vi "create_control.vi"(6 "wait for reply (T)":bool=TRUE, 7 "constant":bool, 8 "error in":errorcluster, 9 "terminal_index":i32, 10 "object_id":i32) -> (0 "error out":errorcluster, 1 "timed out?":bool, 3 "created_object_id":i32)   [LabVIEW 2025, in "Scripting Server.lvlib"]
doc: "Creates a control or indicator on the terminal specified by Object ID and Terminal Index, depending on if it's a in- or output of the node. If Constant is set to True, it can only be used on node inputs and will create a constant.\nIt will return the reference to the created control or indicator, that is a reference to the frontpanel element. If constant is True it returns a reference to the block diagram object (constant).\nWhen creating a control or constant you can pass a value to be written to that element."
uses:
  Scripting Server.lvlib
  create_control Argument--cluster.ctl
  create_control (Reply Payload)--cluster.ctl
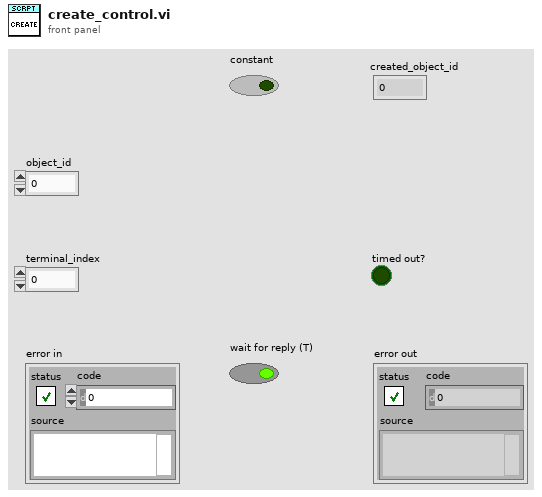
[diagram p1: front panel]
types:
  T1 = typedef "Scripting Server.lvlib/create_control Argument--cluster.ctl" = cluster{"Object ID":i32, "Terminal Index":i32, "Constant":bool, "Wait Notifier":refnum<notifier>, "wait for reply":bool, "Value":string}
  T2 = typedef "Scripting Server.lvlib/Request Events--cluster.ctl" = cluster{"Stop Module":refnum<user-event>, "Show Panel":refnum<user-event>, "Hide Panel":refnum<user-event>, "Get Module Execution Status":refnum<user-event>, "Show Diagram":refnum<user-event>, "New VI":refnum<user-event>, "Add Object":refnum<user-event>, "Connect Objects":refnum<user-event>, "Get Object Terminals":refnum<user-event>, "get vi error list":refnum<user-event>, "Cleanup VI":refnum<user-event>, "create_control":refnum<user-event>, "Run VI":refnum<user-event>, "add_to_selection":refnum<user-event>, "clear_selection_list":refnum<user-event>, "remove_from_selection":refnum<user-event>, "enclose_selection":refnum<user-event>}
  T3 = typedef "Scripting Server.lvlib/create_control (Reply Payload)--cluster.ctl" = cluster{"Object ID":i32, "error":errorcluster}
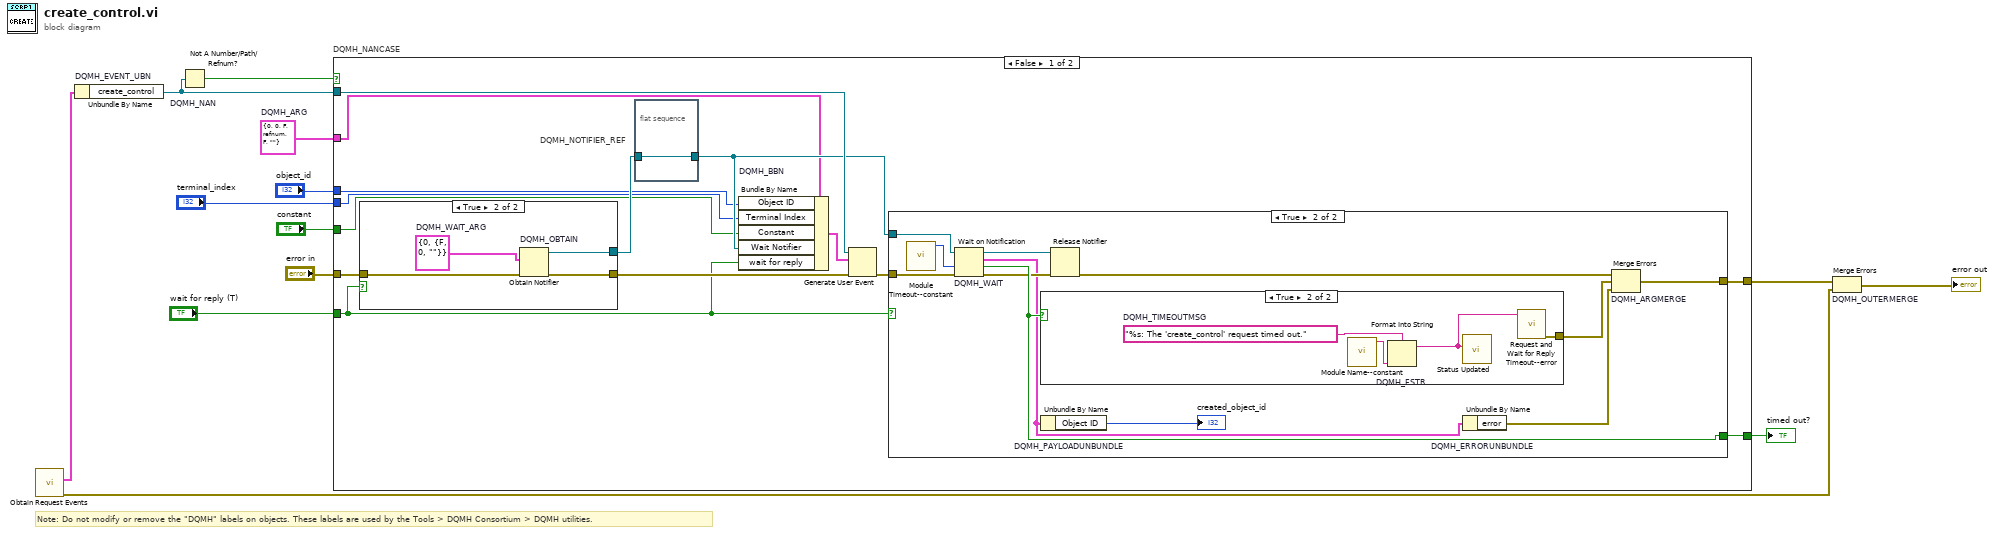
[diagram p0: block diagram]
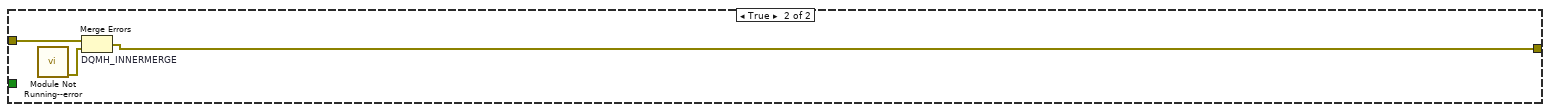
[diagram p5: hidden frame]
diagram:
  w7 = T1 {"Object ID"=0, "Terminal Index"=0, "Constant"=FALSE, "Wait Notifier"=refnum, "wait for reply"=FALSE, "Value"=""}  # DQMH_ARG
  # "Note: Do not modify or remove the \"DQMH\" labels on objects. These labels are used by the Tools > DQMH Consortium > DQMH utilities."
  n1 = call "Obtain Request Events.vi"() -> ("error out"=w2:errorcluster, "Scripting Server Request Events"=w1:T2)  [unwired: 10 in]
  n2 = Unbundle By Name "DQMH_EVENT_UBN"(w1) -> ("create_control"=w11:refnum<user-event>)
  n3 = Not A Number/Path/Refnum? "DQMH_NAN"(number/path/refnum=w11) -> (NaN/Path/Refnum?=w10:bool)
  n4 = case "DQMH_NANCASE" shown="False" w10 {
    tunnel: "error in" -> [w27 w53]
    tunnel: w11 -> [w25 _]
    tunnel: [w22 w52] -> w8
    tunnel: [w23 _] -> w9
    tunnel: w7 -> [w18 _]
    tunnel: "object_id" -> [w17 _]
    tunnel: "terminal_index" -> [w16 _]
    tunnel: "constant" -> [w15 _]
    tunnel: "wait for reply (T)" -> [w14 _]
    frame False {
      n5 = case shown="True" w14 {
        tunnel: w27 -> [w46 w50]
        tunnel: [w46 w49] -> w24
        tunnel: [_ w47] -> w20
        frame False {
        }
        frame True {
          w48 = T3 {"Object ID"=0, "error"={"status"=FALSE, "code"=0, "source"=""}}  # DQMH_WAIT_ARG
          n6 = Obtain Notifier "DQMH_OBTAIN"(notification data type=w48, error in (no error)=w50) -> (notifier out=w47:refnum<notifier>, error out=w49:errorcluster)  [unwired: 2 in, 1 out]
        }
      }
      n7 = flat-sequence "DQMH_NOTIFIER_REF" {
        tunnel: w20 -> [w28]
        tunnel: [w28] -> w19
        frame #0 {
        }
      }
      n8 = Bundle By Name "DQMH_BBN"(cluster=w18, "Object ID"=w17, "Terminal Index"=w16, "Constant"=w15, "Wait Notifier"=w19, "wait for reply"=w14) -> (w21:T1)
      n9 = Generate User Event(user event=w25, event data cluster=w21, error in=w24) -> (error out=w26:errorcluster)  [unwired: 1 in, 1 out]
      n10 = case shown="True" w14 {
        tunnel: w26 -> [w29 w41]
        tunnel: w19 -> [_ w40]
        tunnel: [_ w38] -> w23
        tunnel: [w29 w37] -> w22
        frame False {
        }
        frame True {
          n11 = call "Module Timeout--constant.vi"() -> ("Module Timeout"=w31:i32)  [unwired: 11 in]
          n12 = Wait on Notification "DQMH_WAIT"(notifier=w40, timeout in ms (-1)=w31, error in (no error)=w41) -> (notifier out=w39:refnum<notifier>, notification=w32:T3, timed out?=w38:bool, error out=w36:errorcluster)  [unwired: 1 in]
          n13 = case shown="True" w38 {
            tunnel: [_ w43] -> w33
            frame False {
            }
            frame True {
              w45 = "%s: The 'create_control' request timed out."  # DQMH_TIMEOUTMSG
              n14 = call "Module Name--constant.vi"() -> ("Module Name"=w42:string)  [unwired: 11 in]
              n15 = Format Into String "DQMH_FSTR"(format string=w45, w42) -> (resulting string=w44:string)  [unwired: 2 in, 1 out]
              n16 = call "Status Updated.vi"("Status"=w44) -> ()  [unwired: 10 in, 1 out]
              n17 = call "Request and Wait for Reply Timeout--error.vi"("Error Message"=w44) -> ("error out"=w43:errorcluster)  [unwired: 10 in]
            }
          }
          n18 = Unbundle By Name "DQMH_PAYLOADUNBUNDLE"(w32) -> ("Object ID"=→"created_object_id":i32)
          n19 = Release Notifier(notifier=w39, error in (no error)=w36) -> (error out=w35:errorcluster)  [unwired: 1 in, 2 out]
          n20 = Unbundle By Name "DQMH_ERRORUNBUNDLE"(w32) -> ("error"=w34:errorcluster)
          n21 = Merge Errors "DQMH_ARGMERGE"(w35, w33, w34) -> (w37:errorcluster)
        }
      }
    }
    frame True {
      n22 = call "Module Not Running--error.vi"() -> ("error out"=w51:errorcluster)  [unwired: 11 in]
      n23 = Merge Errors "DQMH_INNERMERGE"(w53, w51) -> (w52:errorcluster)
    }
  }
  "timed out?" <- w9
  n24 = Merge Errors "DQMH_OUTERMERGE"(w8, w2) -> (→"error out":errorcluster)
